vi "PVCAM_CheckStatus.vi"(8 "error in (no error)":errorcluster, 11 "hCam":i16) -> (0 "error out":errorcluster, 2 "bytes_remaining":u32, 3 "status":i16)   [LabVIEW 2021]
uses:
  pvcam64.dll
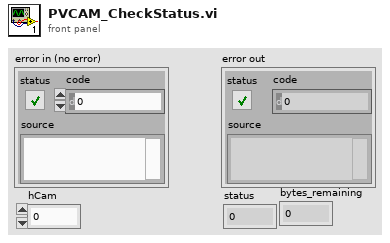
[diagram p1: front panel]
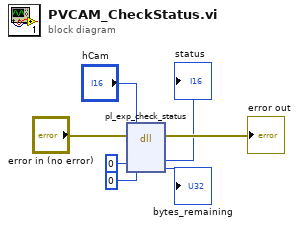
[diagram p0: block diagram]
diagram:
  n1 = dll-call lib="pvcam64.dll" fn="pl_exp_check_status"(error in="error in (no error)", "hCam"="hCam", "status"=i16 0, "bytes_remaining"=u32 0) -> (error out=→"error out":errorcluster, "status"=→"status":i16, "bytes_remaining"=→"bytes_remaining":u32)  [unwired: 4 in, 1 out]
